vi "RandomState.vi"(11 "Field Geometry":dbl[](array[numeric])) -> (3 "Array":dbl[](array[numeric]))   [LabVIEW 2018]
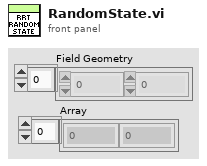
[diagram p1: front panel]
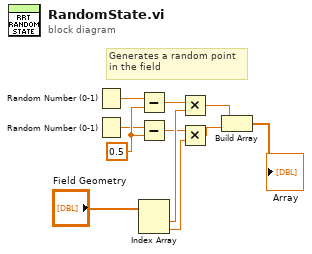
[diagram p0: block diagram]
diagram:
  w6 = 0.5 ("y")
  # "Generates a random point\nin the field"
  n1 = Random Number (0-1)() -> (number: 0 to 1=w4:dbl)
  n2 = Random Number (0-1)() -> (number: 0 to 1=w5:dbl)
  n3 = Subtract(x=w4, y=w6) -> (x-y=w7:dbl)
  n4 = Subtract(x=w5, y=w6) -> (x-y=w8:dbl)
  n5 = Index Array(array="Field Geometry") -> (element #1=w9:dbl, element #2=w10:dbl)  [unwired: 2 in]
  n6 = Multiply(x=w7, y=w9) -> (x*y=w2:dbl)
  n7 = Multiply(x=w8, y=w10) -> (x*y=w3:dbl)
  n8 = Build Array(w2, w3) -> (→"Array":dbl[])
